vi "set_number_of_pulses.vi"(8 "error in (no error)":errorcluster, 10 "number of pulses":i64, 11 "GenericClock.lvclass in":refnum<class "GenericClock.lvclass">) -> (0 "error out":errorcluster, 3 "GenericClock.lvclass out":refnum<class "GenericClock.lvclass">)   [LabVIEW 2010, in "GenericClock.lvclass"]
uses:
  GenericClock.lvclass
  GenericClock.lvclass/GenericClock.ctl
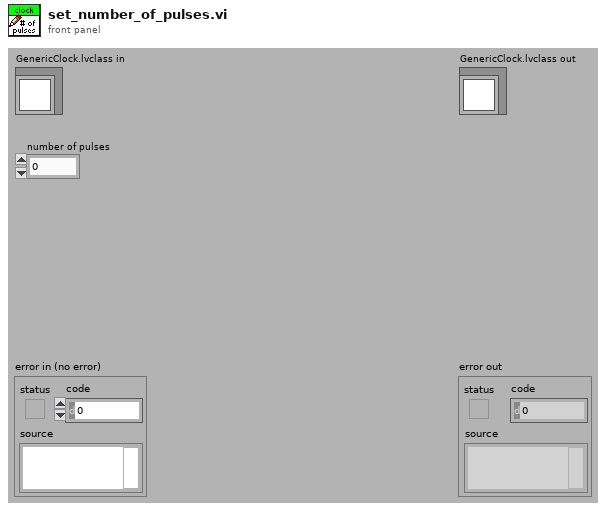
[diagram p1: front panel]
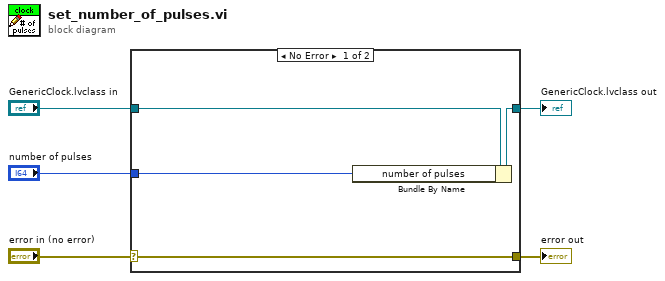
[diagram p0: block diagram]
diagram:
  n1 = case shown="No Error" "error in (no error)" {
    selector: "error in (no error)" -> [w9 w10]
    tunnel: [w9 w10] -> w4
    tunnel: [w7 w11] -> w2
    tunnel: "GenericClock.lvclass in" -> [w8 w11]
    tunnel: "number of pulses" -> [w6 _]
    frame No Error {
      n2 = Bundle By Name(cluster=w8, "number of pulses"=w6) -> (w7:refnum<class "GenericClock.lvclass">)
    }
    frame Error {
    }
  }
  "error out" <- w4
  "GenericClock.lvclass out" <- w2
